vi "File Info Test.vi"(11 "Error In":errorcluster) -> (15 "Error Out":errorcluster)   [LabVIEW 2021, in "Test Files.lvlib"]
doc: "This VI has the test cases for checking the file information obtained from FileInfo.vi"
uses:
  Test Files.lvlib
  CustomSortPath.lvlib
  <vilib>/addons/_JKI Toolkits/Caraya/classes/Test/Test.lvclass
  <vilib>/addons/_JKI Toolkits/Caraya/classes/Assert/Assert.lvclass
  <vilib>/addons/_JKI Toolkits/Caraya/classes/Assert/Assert Equal Value_Variant.vi
panel:
  # "File/Folder Information Test"
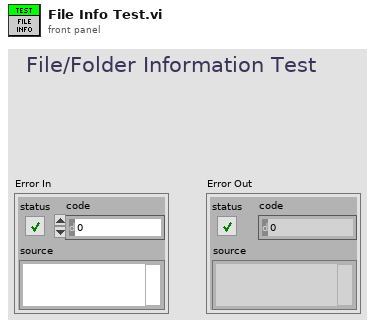
[diagram p1: front panel]
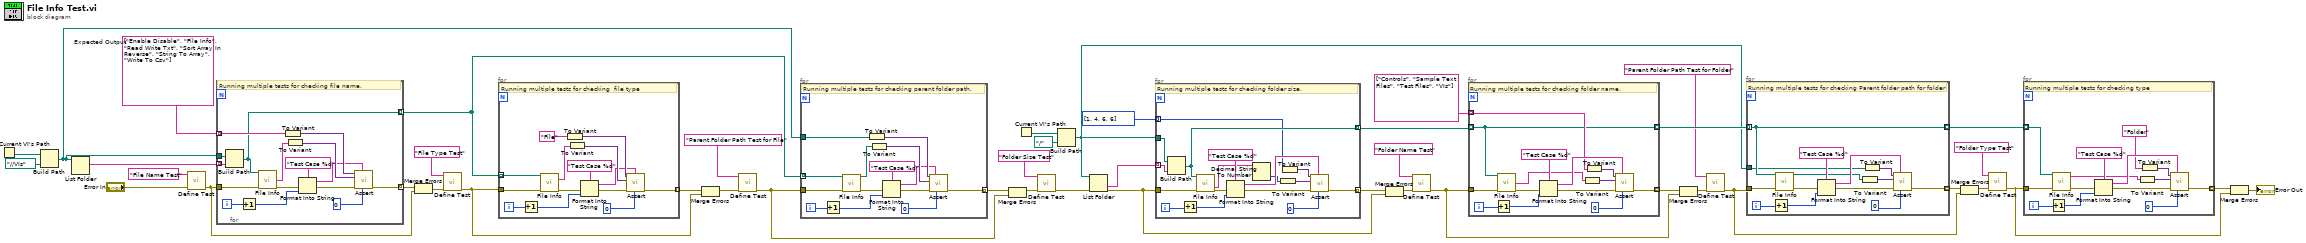
[diagram p0: block diagram]
diagram:
  w42 = string[] ["Enable Disable", "File Info", "Read Write Txt", "Sort Array In Reverse", "String To Array", "Write To Csv"]  # Expected Output
  n1 = Current VI's Path() -> (path=w45:path)
  n2 = Build Path(base path=w45, name or relative path=path "../../VIs") -> (appended path=w24:path)
  n3 = List Folder(path=w24) -> (filenames=w23:string[])  [unwired: 3 in, 3 out]
  n4 = call <vilib>:"Define Test.vi"("error in (no error)"="Error In", "Label (VI Title)"="File Name Test") -> ("error out"=w19:errorcluster)  [unwired: 8 in, 1 out]
  n5 = for {
    tunnel: w42 -> [w55] mode=indexing
    tunnel: w24 -> [w49]
    tunnel: w23 -> [w48] mode=indexing
    tunnel: [w47] -> w22 mode=indexing
    tunnel: w19 -> [w61]
    tunnel: [w57] -> w20 mode=indexing
    i -> [w54]
    # "Running multiple tests for checking file name."
    n6 = Build Path(base path=w49, name or relative path=w48) -> (appended path=w47:path)
    n7 = Increment(x=w54) -> (x+1=w51:i32)
    n8 = call "File Info.vi"("File/Folder Path"=w47, "error in (no error)"=w61) -> ("Name"=w56:string, "error out"=w60:errorcluster)  [unwired: 9 in, 3 out]
    n9 = To Variant(anything=w55) -> (Variant=w58:variant)
    n10 = To Variant(anything=w56) -> (Variant=w59:variant)
    n11 = Format Into String(format string="Test Case %d", error in=w60, w51) -> (resulting string=w50:string, error out=w53:errorcluster)  [unwired: 1 in]
    n12 = call-poly <vilib>:"Assert.vi"("error code (1)"=0, "Label"=w50, "error in (no error)"=w53, "Y"=w59, "X"=w58) -> ("error out"=w57:errorcluster)  [unwired: 5 in, 1 out]
  }
  n13 = Merge Errors(w20, w19) -> (w21:errorcluster)
  n14 = call <vilib>:"Define Test.vi"("error in (no error)"=w21, "Label (VI Title)"="File Type Test") -> ("error out"=w17:errorcluster)  [unwired: 8 in, 1 out]
  n15 = for {
    tunnel: w22 -> [w64] mode=indexing
    tunnel: w17 -> [w75]
    tunnel: [w71] -> w18 mode=indexing
    i -> [w70]
    # "Running multiple tests for checking  file type"
    n16 = Increment(x=w70) -> (x+1=w67:i32)
    n17 = call "File Info.vi"("File/Folder Path"=w64, "error in (no error)"=w75) -> ("Type"=w66:string, "error out"=w74:errorcluster)  [unwired: 9 in, 3 out]
    n18 = To Variant(anything="File" ("Type")) -> (Variant=w72:variant)
    n19 = To Variant(anything=w66) -> (Variant=w73:variant)
    n20 = Format Into String(format string="Test Case %d", error in=w74, w67) -> (resulting string=w63:string, error out=w69:errorcluster)  [unwired: 1 in]
    n21 = call-poly <vilib>:"Assert.vi"("error code (1)"=0, "Label"=w63, "error in (no error)"=w69, "Y"=w73, "X"=w72) -> ("error out"=w71:errorcluster)  [unwired: 5 in, 1 out]
  }
  n22 = Merge Errors(w18, w17) -> (w16:errorcluster)
  n23 = call <vilib>:"Define Test.vi"("error in (no error)"=w16, "Label (VI Title)"="Parent Folder Path Test for File") -> ("error out"=w13:errorcluster)  [unwired: 8 in, 1 out]
  n24 = for {
    tunnel: w22 -> [w80] mode=indexing
    tunnel: w24 -> [w79]
    tunnel: w13 -> [w89]
    tunnel: [w85] -> w14 mode=indexing
    i -> [w84]
    # "Running multiple tests for checking parent folder path."
    n25 = Increment(x=w84) -> (x+1=w81:i32)
    n26 = call "File Info.vi"("File/Folder Path"=w80, "error in (no error)"=w89) -> ("ParentFolderPath"=w78:path, "error out"=w88:errorcluster)  [unwired: 9 in, 3 out]
    n27 = To Variant(anything=w79) -> (Variant=w86:variant)
    n28 = To Variant(anything=w78) -> (Variant=w87:variant)
    n29 = Format Into String(format string="Test Case %d", error in=w88, w81) -> (resulting string=w77:string, error out=w83:errorcluster)  [unwired: 1 in]
    n30 = call-poly <vilib>:"Assert.vi"("error code (1)"=0, "Label"=w77, "error in (no error)"=w83, "Y"=w87, "X"=w86) -> ("error out"=w85:errorcluster)  [unwired: 5 in, 1 out]
  }
  n31 = Merge Errors(w14, w13) -> (w15:errorcluster)
  n32 = Current VI's Path() -> (path=w37:path)
  n33 = call <vilib>:"Define Test.vi"("error in (no error)"=w15, "Label (VI Title)"="Folder Size Test") -> ("error out"=w34:errorcluster)  [unwired: 8 in, 1 out]
  n34 = Build Path(base path=w37, name or relative path=path "../..") -> (appended path=w25:path)
  n35 = List Folder(path=w25, error in=w34) -> (folder names=w36:string[], error out=w10:errorcluster)  [unwired: 2 in, 2 out]
  n36 = for {
    tunnel: [w104] -> w31 mode=indexing
    tunnel: w36 -> [w95] mode=indexing
    tunnel: w25 -> [w96]
    tunnel: i64[] [1, 4, 6, 6] ("number") -> [w94] mode=indexing
    tunnel: w10 -> [w106]
    tunnel: [w103] -> w11 mode=indexing
    i -> [w101]
    # "Running multiple tests for checking folder size."
    n37 = Build Path(base path=w96, name or relative path=w95) -> (appended path=w104:path)
    n38 = Increment(x=w101) -> (x+1=w100:i32)
    n39 = call "File Info.vi"("File/Folder Path"=w104, "error in (no error)"=w106) -> ("Size"=w98:string, "error out"=w105:errorcluster)  [unwired: 9 in, 3 out]
    n40 = Format Into String(format string="Test Case %d", error in=w105, w100) -> (resulting string=w97:string, error out=w102:errorcluster)  [unwired: 1 in]
    n41 = Decimal String To Number(string=w98) -> (number=w93:i32)  [unwired: 2 in, 1 out]
    n42 = To Variant(anything=w93) -> (Variant=w92:variant)
    n43 = To Variant(anything=w94) -> (Variant=w91:variant)
    n44 = call-poly <vilib>:"Assert.vi"("error code (1)"=0, "Label"=w97, "error in (no error)"=w102, "Y"=w92, "X"=w91) -> ("error out"=w103:errorcluster)  [unwired: 5 in, 1 out]
  }
  n45 = Merge Errors(w11, w10) -> (w12:errorcluster)
  n46 = call <vilib>:"Define Test.vi"("error in (no error)"=w12, "Label (VI Title)"="Folder Name Test") -> ("error out"=w7:errorcluster)  [unwired: 8 in, 1 out]
  n47 = for {
    tunnel: string[] ["Controls", "Sample Text Files", "Test Files", "VIs"] -> [w110] mode=indexing
    tunnel: w31 -> [w108] mode=indexing
    tunnel: [w108] -> w29 mode=indexing
    tunnel: w7 -> [w120]
    tunnel: [w116] -> w9 mode=indexing
    i -> [w114]
    # "Running multiple tests for checking folder name."
    n48 = Increment(x=w114) -> (x+1=w113:i32)
    n49 = call "File Info.vi"("File/Folder Path"=w108, "error in (no error)"=w120) -> ("Name"=w109:string, "error out"=w119:errorcluster)  [unwired: 9 in, 3 out]
    n50 = Format Into String(format string="Test Case %d", error in=w119, w113) -> (resulting string=w111:string, error out=w115:errorcluster)  [unwired: 1 in]
    n51 = To Variant(anything=w109) -> (Variant=w118:variant)
    n52 = To Variant(anything=w110) -> (Variant=w117:variant)
    n53 = call-poly <vilib>:"Assert.vi"("error code (1)"=0, "Label"=w111, "error in (no error)"=w115, "Y"=w118, "X"=w117) -> ("error out"=w116:errorcluster)  [unwired: 5 in, 1 out]
  }
  n54 = Merge Errors(w9, w7) -> (w8:errorcluster)
  n55 = call <vilib>:"Define Test.vi"("error in (no error)"=w8, "Label (VI Title)"="Parent Folder Path Test for Folder") -> ("error out"=w4:errorcluster)  [unwired: 8 in, 1 out]
  n56 = for {
    tunnel: w29 -> [w124] mode=indexing
    tunnel: [w124] -> w27 mode=indexing
    tunnel: w25 -> [w122]
    tunnel: w4 -> [w134]
    tunnel: [w130] -> w5 mode=indexing
    i -> [w128]
    # "Running multiple tests for checking Parent folder path for folder"
    n57 = Increment(x=w128) -> (x+1=w127:i32)
    n58 = call "File Info.vi"("File/Folder Path"=w124, "error in (no error)"=w134) -> ("ParentFolderPath"=w123:path, "error out"=w133:errorcluster)  [unwired: 9 in, 3 out]
    n59 = Format Into String(format string="Test Case %d", error in=w133, w127) -> (resulting string=w125:string, error out=w129:errorcluster)  [unwired: 1 in]
    n60 = To Variant(anything=w123) -> (Variant=w132:variant)
    n61 = To Variant(anything=w122) -> (Variant=w131:variant)
    n62 = call-poly <vilib>:"Assert.vi"("error code (1)"=0, "Label"=w125, "error in (no error)"=w129, "Y"=w132, "X"=w131) -> ("error out"=w130:errorcluster)  [unwired: 5 in, 1 out]
  }
  n63 = Merge Errors(w5, w4) -> (w6:errorcluster)
  n64 = call <vilib>:"Define Test.vi"("error in (no error)"=w6, "Label (VI Title)"="Folder Type Test") -> ("error out"=w1:errorcluster)  [unwired: 8 in, 1 out]
  n65 = for {
    tunnel: w27 -> [w138] mode=indexing
    tunnel: w1 -> [w148]
    tunnel: [w144] -> w3 mode=indexing
    i -> [w142]
    # "Running multiple tests for checking type"
    n66 = Increment(x=w142) -> (x+1=w141:i32)
    n67 = call "File Info.vi"("File/Folder Path"=w138, "error in (no error)"=w148) -> ("Type"=w136:string, "error out"=w147:errorcluster)  [unwired: 9 in, 3 out]
    n68 = Format Into String(format string="Test Case %d", error in=w147, w141) -> (resulting string=w139:string, error out=w143:errorcluster)  [unwired: 1 in]
    n69 = To Variant(anything=w136) -> (Variant=w146:variant)
    n70 = To Variant(anything="Folder" ("format string")) -> (Variant=w145:variant)
    n71 = call-poly <vilib>:"Assert.vi"("error code (1)"=0, "Label"=w139, "error in (no error)"=w143, "Y"=w146, "X"=w145) -> ("error out"=w144:errorcluster)  [unwired: 5 in, 1 out]
  }
  n72 = Merge Errors(w3, w1) -> (→"Error Out":errorcluster)
